vi "Rotor sweep.vi"() -> ()   [LabVIEW 2012]
panel:
  in  ".NET Container":refnum<k24>(container)
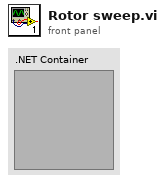
[diagram p1: front panel]
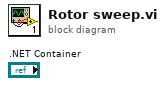
[diagram p0: block diagram]
diagram:
